vi "Update-temperature-variables.vi"(8 "error in":errorcluster, 11 "Data ref. in":refnum<data-value>) -> (0 "error IO":errorcluster, 3 "Data ref.":refnum<data-value>)   [LabVIEW 2013, in "CameraVision.lvlib" / "CV-Main.lvclass"]
doc: "If the 'Temperature field' option is enabled, this function loads the temperature field regression file into memory. The file is obtained from '<Application>\\Program data\\temperatureFieldRegression.dat'.\nThe regression file provides the data for a linear piecewise approximation of the temperature [°C] versus intensity ratio [-] function. This function must be generated beforehand based on the specific hardware used (f-Theta lense, mirror system, dichroic mirror, filters, camera sensitivity).\n\nThis function also corrects the regression data for differences in the exposure time between the two cameras. It also linearizes the intensity in case the lin-log camera exposure mode is used."
uses:
  CV-Main.lvclass
  CV-Main.lvclass/CV-Main.ctl
  Read Temperature params.vi
  Read Acquis params.vi
  Read Storage params.vi
  Temperature/CV-Temperature.lvclass
  Acquisition/CV-Acquisition.lvclass
  Storage/CV-Storage.lvclass
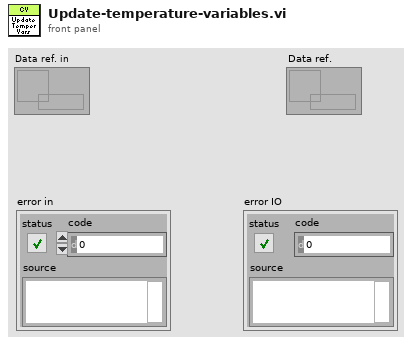
[diagram p1: front panel]
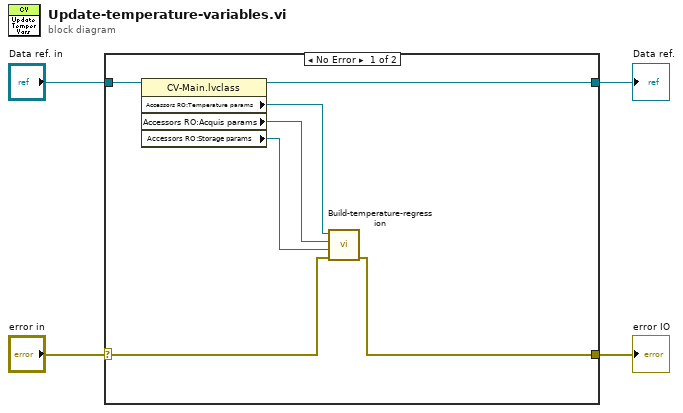
[diagram p0: block diagram]
diagram:
  n1 = case shown="No Error" "error in" {
    selector: "error in" -> [w10 w13]
    tunnel: [w11 w13] -> w4
    tunnel: "Data ref. in" -> [w9 w12]
    tunnel: [w8 w12] -> w1
    frame No Error {
      n2 = property class="CV-Main.lvclass"(reference=w9) -> (reference out=w8:refnum<data-value>, "Accessors RO:Temperature params"=w7:refnum<data-value>, "Accessors RO:Acquis params"=w6:refnum<data-value>, "Accessors RO:Storage params"=w5:refnum<data-value>)  [unwired: 1 in, 1 out]
      n3 = call "Build-temperature-regression.vi"("error in (no error)"=w10, "Storage params in"=w5, "Acquis. params in"=w6, "Temperature params in"=w7) -> ("error out"=w11:errorcluster)  [unwired: 4 in, 3 out]
    }
    frame Error {
    }
  }
  "error IO" <- w4
  "Data ref." <- w1
